vi "Get Picture.vi"(8 "error in (no error)":errorcluster, 11 "Plastic Parts in":refnum<class "Plastic Parts.lvclass">) -> (0 "error out":errorcluster, 2 "Picture":picture, 3 "Plastic Parts out":refnum<class "Plastic Parts.lvclass">)   [LabVIEW 2020, in "Plastic Parts.lvclass"]
uses:
  Plastic Parts.lvclass
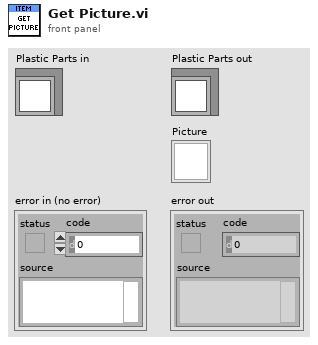
[diagram p1: front panel]
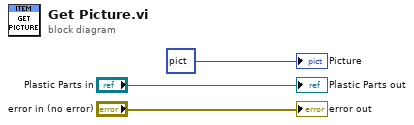
[diagram p0: block diagram]
diagram:
  "error out" <- "error in (no error)"
  "Plastic Parts out" <- "Plastic Parts in"
  "Picture" <- picture bytes[3230] ("new picture")
